vi "Save New Class.vi"(8 "error in (no error)":errorcluster, 11 "QControl Creation in":refnum<class "QControl Creation.lvclass">) -> (0 "error out":errorcluster, 2 "New LVClassLibrary out":refnum<vi>, 3 "QControl Creation out":refnum<class "QControl Creation.lvclass">)   [LabVIEW 2015, in "QControl Creation.lvclass"]
doc: "<b> </b> <b> </b>\n©2016 Q Software Innovations, LLC (QSI)\nwritten by Quentin Alldredge\nproduced in LabVIEW 2015\n\nsupport@qsoftwareinnovations.com\nwww.qsoftwareinnovations.com\n\nAll rights reserved.\n\nRedistribution and use in source and binary forms, with or without modification, are permitted provided that the following conditions are met:\n\n * Redistributions of source code must retain the above copyright notice, this list of conditions and the following disclaimer.\n * Redistributions in binary form must reproduce the above copyright notice, this list of conditions and the following disclaimer in the documentation and/or other materials provided with the distribution.\n * Neither the name of Q Software Innovations, LLC. nor the names of its contributors may be used to endorse or promote products derived from this software without specific prior written permission.\n\nTHIS SOFTWARE IS PROVIDED BY THE COPYRIGHT HOLDERS AND CONTRIBUTORS \"AS IS\" AND ANY EXPRESS OR IMPLIED WARRANTIES, INCLUDING, BUT NOT LIMITED TO, THE IMPLIED WARRANTIES OF MERCHANTABILITY AND FITNESS FOR A PARTICULAR PURPOSE ARE DISCLAIMED. IN NO EVENT SHALL THE COPYRIGHT OWNER OR CONTRIBUTORS BE LIABLE FOR ANY DIRECT, INDIRECT, INCIDENTAL, SPECIAL, EXEMPLARY, OR CONSEQUENTIAL DAMAGES (INCLUDING, BUT NOT LIMITED TO, PROCUREMENT OF SUBSTITUTE GOODS OR SERVICES; LOSS OF USE, DATA, OR PROFITS; OR BUSINESS INTERRUPTION) HOWEVER CAUSED AND ON ANY THEORY OF LIABILITY, WHETHER IN CONTRACT, STRICT LIABILITY, OR TORT (INCLUDING NEGLIGENCE OR OTHERWISE) ARISING IN ANY WAY OUT OF THE USE OF THIS SOFTWARE, EVEN IF ADVISED OF THE POSSIBILITY OF SUCH DAMAGE."
uses:
  QControl Creation.lvclass
  QControl Creation.lvclass/QControl Creation.ctl
  New QControl Info/New QControl Info.lvclass/New QControl Info.ctl
  New QControl Info/Read New Class Path.vi
  New QControl Info/Read App Refnum.vi
  <vilib>/Utility/error.llb/Error Cluster From Error Code.vi
  <vilib>/ErrorRing/Error Ring.xnode
  New QControl Info/New QControl Info.lvclass
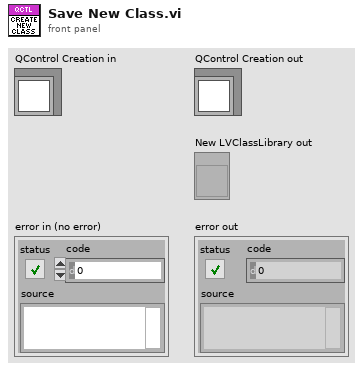
[diagram p1: front panel]
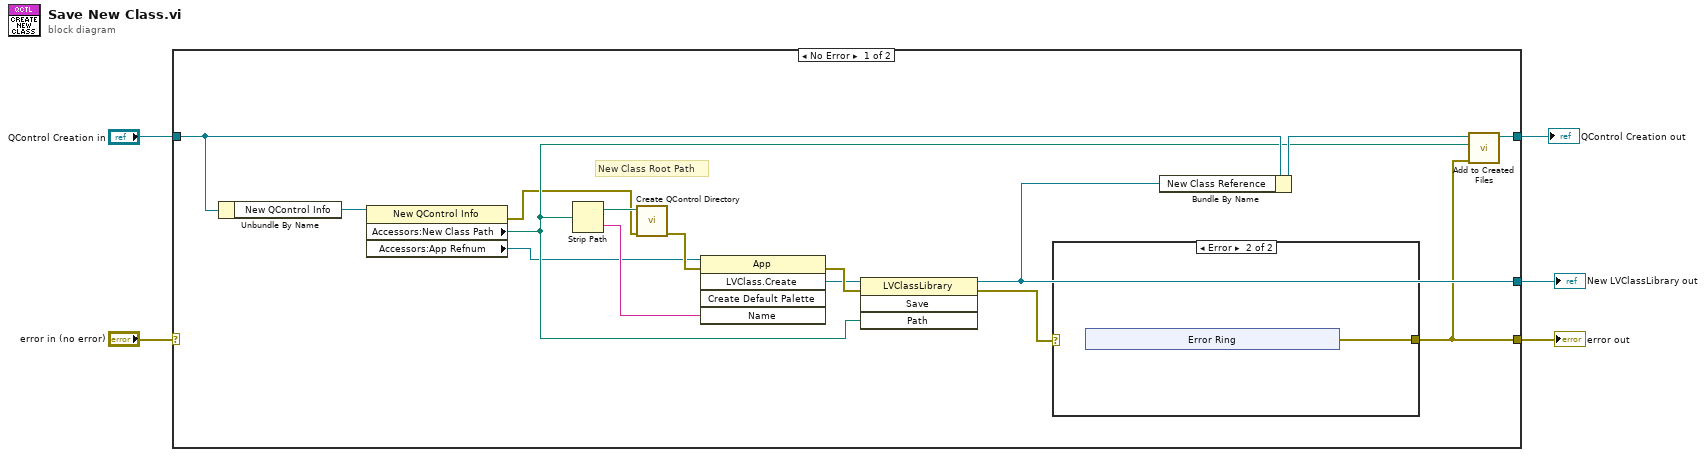
[diagram p0: block diagram]
diagram:
  n1 = case shown="No Error" "error in (no error)" {
    selector: "error in (no error)" -> [_ w29]
    tunnel: [w20 _] -> w4
    tunnel: [w11 w29] -> w3
    tunnel: "QControl Creation in" -> [w14 w28]
    tunnel: [w12 w28] -> w1
    frame No Error {
      # "New Class Root Path"
      n2 = Unbundle By Name(w14) -> ("New QControl Info"=w10:refnum<data-value>)
      n3 = property class="New QControl Info"(reference=w10) -> (error out=w6:errorcluster, "Accessors:New Class Path"=w8:path, "Accessors:App Refnum"=w7:refnum<vi>)  [unwired: 1 in, 1 out]
      n4 = Strip Path(path=w8) -> (stripped path=w9:path, name=w19:string)
      n5 = call "Create QControl Directory.vi"("Error In"=w6, "Path"=w9) -> ("Error Out"=w17:errorcluster)  [unwired: 8 in, 1 out]
      n6 = invoke class="App" method="LVClass.Create"(reference=w7, error in=w17, "Name"=w19) -> (error out=w18:errorcluster, "LVClass.Create"=w16:refnum<vi>)  [unwired: 2 in, 3 out]
      n7 = invoke class="LVClassLibrary" method="Save"(reference=w16, error in=w18, "Path"=w8) -> (reference out=w20:refnum<vi>, error out=w15:errorcluster)  [unwired: 1 in, 2 out]
      n8 = case shown="Error" w15 {
        selector: w15 -> [w21 _]
        tunnel: [w21 w22] -> w11
        frame No Error {
        }
        frame Error {
          n9 = xnode "Error Ring"() -> ("error out"=w22:errorcluster)
        }
      }
      n10 = Bundle By Name(cluster=w14, "New Class Reference"=w20) -> (w13:refnum<class "QControl Creation.lvclass">)
      n11 = call "Add to Created Files.vi"("error in (no error)"=w11, "Path to Add"=w8, "QControl Creation in"=w13) -> ("QControl Creation out"=w12:refnum<class "QControl Creation.lvclass">)  [unwired: 8 in]
    }
    frame Error {
    }
  }
  "New LVClassLibrary out" <- w4
  "error out" <- w3
  "QControl Creation out" <- w1
